vi "Convert Boolean to Disabled Enum.vi"(11 "Enabled?":bool) -> (3 "Disabled Enum":T1(ring))   [LabVIEW 2020, in "MacroAssert.lvlib"]
doc: "Outputs Enabled if the input is TRUE, and Disabled and Grayed Out if the input is FALSE."
uses:
  MacroAssert.lvlib
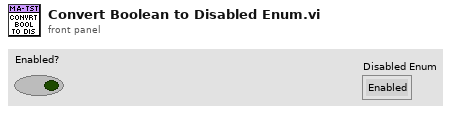
[diagram p1: front panel]
types:
  T1 = enum8{"Enabled", "Disabled", "Disabled and Grayed Out"}
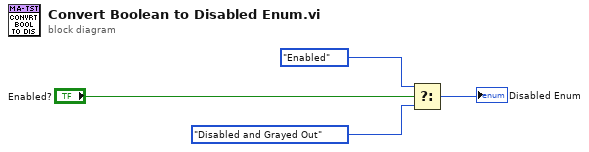
[diagram p0: block diagram]
diagram:
  n1 = Select(t=T1."Enabled" ("Disabled"), s="Enabled?", f=T1."Disabled and Grayed Out" ("Disabled")) -> (s? t:f=→"Disabled Enum":T1)
